vi "Insert Test Step.vi"(8 "error in (no error)":errorcluster, 10 "Insert Test Step":T1, 11 "Test Executive Builder Model in":refnum<class "Test Executive Builder Model.lvclass">) -> (0 "error out":errorcluster, 3 "Test Executive Builder Model out":refnum<class "Test Executive Builder Model.lvclass">, 5 "Unique ID out":string)   [LabVIEW 2019, in "Test Executive Builder Model.lvclass"]
uses:
  <vilib>/gpm_packages/@cs/Test-executive-builder/Source/Test Executive Builder Model/Test Executive Builder Model/Test Executive Builder Model.lvclass
  C:/Program Files/National Instruments/LabVIEW 2019/vi.lib/ActorFramework/Actor/Actor.lvclass
  <vilib>/gpm_packages/@cs/Test-executive-builder/Source/Application Dependencies/Insert Test Step.ctl
  <vilib>/gpm_packages/@cs/Test-executive-builder/Source/Test Executive Builder Model/Test Executive Builder Model/Test Executive Builder Model.lvclass/Test Executive Builder Model.ctl
  <vilib>/ActorFramework/Actor/Actor.lvclass/Actor.ctl
  <vilib>/ActorFramework/Message Enqueuer/Message Enqueuer.lvclass/Message Enqueuer.ctl
  <vilib>/ActorFramework/Message Enqueuer/Init from Existing Queue.vi
  <vilib>/ActorFramework/Message Enqueuer/Enqueue.vi
  <vilib>/gpm_packages/@cs/Test-executive-builder/Source/Test Executive Builder Model/Test Executive Builder Model Messages/Redraw Tree Msg/Redraw Tree Msg.lvclass
  C:/Program Files/National Instruments/LabVIEW 2019/vi.lib/ActorFramework/Message/Message.lvclass
  <vilib>/ActorFramework/Message Priority Queue/Priority Enqueue.vi
  <vilib>/ActorFramework/Message Enqueuer/Message Enqueuer.lvclass
  <vilib>/gpm_packages/@cs/test-executive/Source/Test Executive/TestExecutive Ref/TestExecutive Ref.lvclass
  <vilib>/gpm_packages/@cs/test-executive/Source/Test Executive/Executioner/Executioner.lvclass
  <vilib>/ActorFramework/Actor/Actor.lvclass
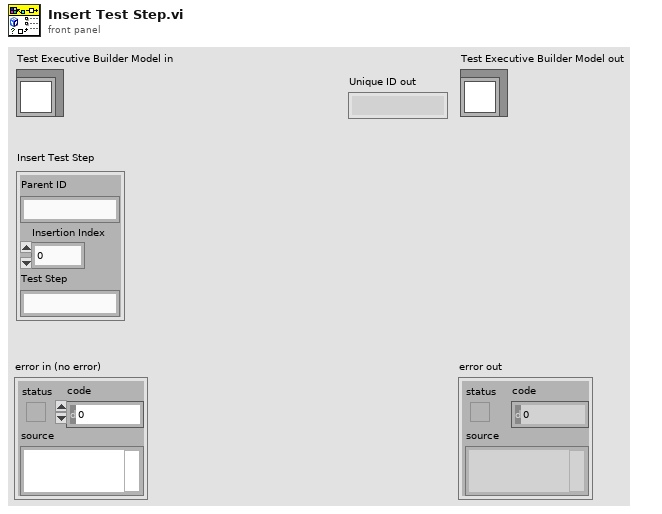
[diagram p1: front panel]
types:
  T1 = typedef "Insert Test Step.ctl" = cluster{"Parent ID":string, "Insertion Index":i32, "Test Step":string}
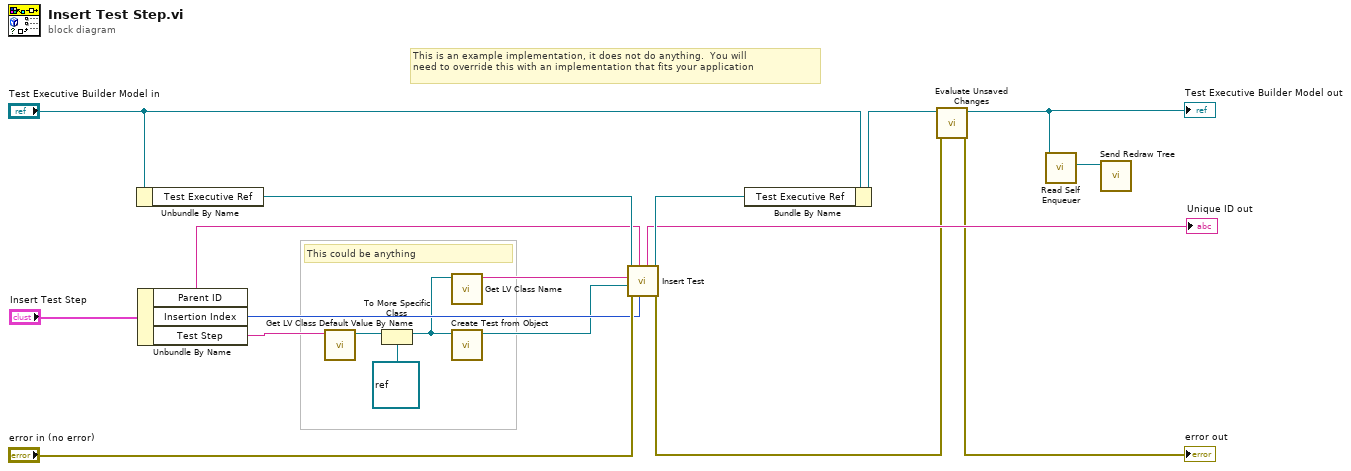
[diagram p0: block diagram]
diagram:
  # "This could be anything"
  # "This is an example implementation, it does not do anything.  You will\nneed to override this with an implementation that fits your application"
  n1 = Unbundle By Name("Test Executive Builder Model in") -> ("Test Executive Ref"=w18:refnum<data-value>)
  n2 = Unbundle By Name("Insert Test Step") -> ("Parent ID"=w14:string, "Insertion Index"=w13:i32, "Test Step"=w12:string)
  n3 = call <vilib>:"Get LV Class Default Value By Name.vi"("class name"=w12) -> ("object"=w11:refnum<class>)  [unwired: 9 in, 1 out]
  n4 = To More Specific Class(target class=refnum<class> refnum, reference=w11) -> (specific class reference=w9:refnum<class>)  [unwired: 1 in, 1 out]
  n5 = call <vilib>:"Get LV Class Name.vi"("object"=w9) -> ("class name"=w8:string)  [unwired: 9 in, 1 out]
  n6 = call <vilib>:"Create Test from Object.vi"("Test"=w9) -> ("Test"=w7:refnum<class "Executioner.lvclass">)  [unwired: 10 in]
  n7 = call <vilib>:"Insert Test.vi"("Insertion Index"=w13, "Parent ID"=w14, "error in (no error)"="error in (no error)", "Test"=w7, "Name"=w8, "Test Executive Ref"=w18) -> ("error out"=w2:errorcluster, "Test Executive Ref out"=w15:refnum<data-value>, "Unique ID out"=→"Unique ID out":string)  [unwired: 2 in, 1 out]
  n8 = Bundle By Name(cluster="Test Executive Builder Model in", "Test Executive Ref"=w15) -> (w4:refnum<class "Test Executive Builder Model.lvclass">)
  n9 = call-dynamic "Evaluate Unsaved Changes.vi"("error in (no error)"=w2, "Test Executive Builder Model in"=w4) -> ("error out"=→"error out":errorcluster, "Test Executive Builder Model out"=w3:refnum<class "Test Executive Builder Model.lvclass">)  [unwired: 8 in]
  "Test Executive Builder Model out" <- w3
  n10 = call <vilib>:"Read Self Enqueuer.vi"("Actor"=w3) -> ("Self Enqueuer"=w5:refnum<class "Message Enqueuer.lvclass">)  [unwired: 10 in]
  n11 = call <vilib>:"Send Redraw Tree.vi"("Message Enqueuer"=w5) -> ()  [unwired: 9 in, 2 out]
